vi "goToStandby.vi"(8 "error in (no error)":errorcluster, 10 "model":refnum<class "Model.lvclass">, 11 "EnabledState in":refnum<class "EnabledState.lvclass">) -> (0 "error out":errorcluster, 2 "model 2":refnum<class "Model.lvclass">, 3 "EnabledState out":refnum<class "EnabledState.lvclass">)   [LabVIEW 2013, in "EnabledState.lvclass"]
uses:
  EnabledState.lvclass
  Model/Model/Model.lvclass
  Typedefs/StateSelector.ctl
  Typedefs/M2AADTTypedefs.lvlib
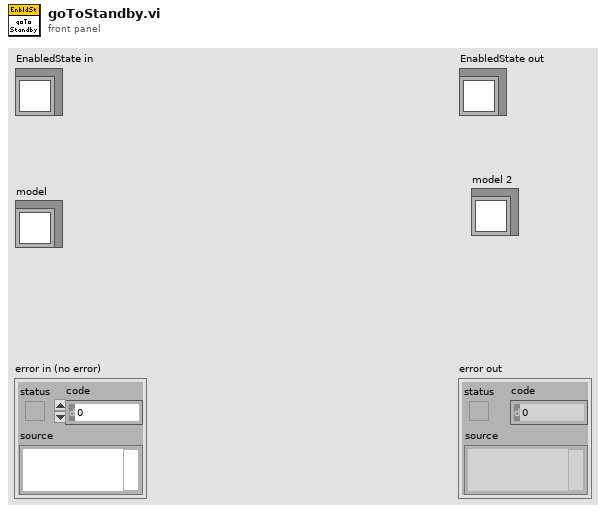
[diagram p1: front panel]
types:
  T1 = typedef "M2AADTTypedefs.lvlib/StateSelector.ctl" = enum16{"EndingCycleState", "FaultState", "InteractiveMotionState", "MovingToNewForceState", "OffState", "PausingState", "StandbyState", "StoppedState"}
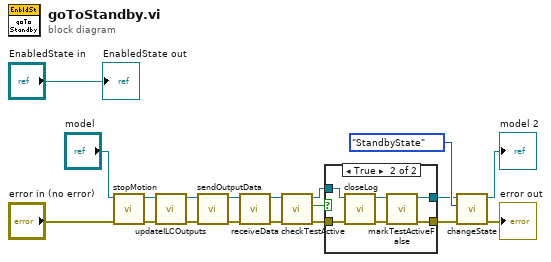
[diagram p0: block diagram]
diagram:
  n1 = call "stopMotion.vi"("error in (no error)"="error in (no error)", "Model in"="model") -> ("error out"=w6:errorcluster, "Model out"=w8:refnum<class "Model.lvclass">)  [unwired: 8 in]
  n2 = call "updateILCOutputs.vi"("error in (no error)"=w6, "Model in"=w8) -> ("error out"=w5:errorcluster, "Model out"=w7:refnum<class "Model.lvclass">)  [unwired: 8 in]
  n3 = call "sendOutputData.vi"("error in (no error)"=w5, "Model in"=w7) -> ("error out"=w2:errorcluster, "Model out"=w4:refnum<class "Model.lvclass">)  [unwired: 8 in]
  n4 = call "receiveData.vi"("error in (no error)"=w2, "Model in"=w4) -> ("error out"=w1:errorcluster, "Model out"=w3:refnum<class "Model.lvclass">)  [unwired: 8 in]
  n5 = call "checkTestActive.vi"("error in (no error)"=w1, "Model in"=w3) -> ("error out"=w11:errorcluster, "testActiveIsTrue"=w13:bool, "Model out"=w12:refnum<class "Model.lvclass">)  [unwired: 7 in]
  n6 = case shown="True" w13 {
    tunnel: [w21 w24] -> w10
    tunnel: [w20 w22] -> w9
    tunnel: w12 -> [w21 w27]
    tunnel: w11 -> [w20 w26]
    frame False {
    }
    frame True {
      n7 = call "closeLog.vi"("error in (no error)"=w26, "Model in"=w27) -> ("error out"=w23:errorcluster, "Model out"=w25:refnum<class "Model.lvclass">)  [unwired: 8 in]
      n8 = call "markTestActiveFalse.vi"("error in (no error)"=w23, "Model in"=w25) -> ("error out"=w22:errorcluster, "Model out"=w24:refnum<class "Model.lvclass">)  [unwired: 8 in]
    }
  }
  n9 = call "changeState.vi"("error in (no error)"=w9, "State:"=StateSelector."StandbyState", "Model in"=w10) -> ("error out"=→"error out":errorcluster, "Model out"=→"model 2":refnum<class "Model.lvclass">)  [unwired: 7 in]
  "EnabledState out" <- "EnabledState in"
